vi "Television.vi"() -> ()   [LabVIEW 2021]
panel:
  in  "Mute":bool
  in  "Volume":dbl(knob) scale=0.0..100.0
  in  "off":bool
  in  "on":bool
  in  "channel2":bool
  in  "channel 1":bool
  in  "WindowsMediaPlayer":refnum<k7>(container)
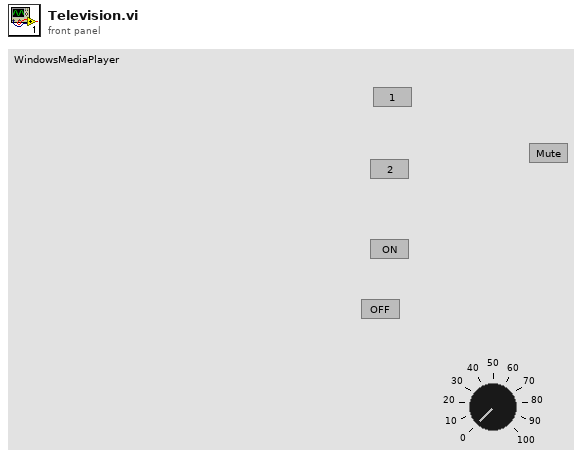
[diagram p1: front panel]
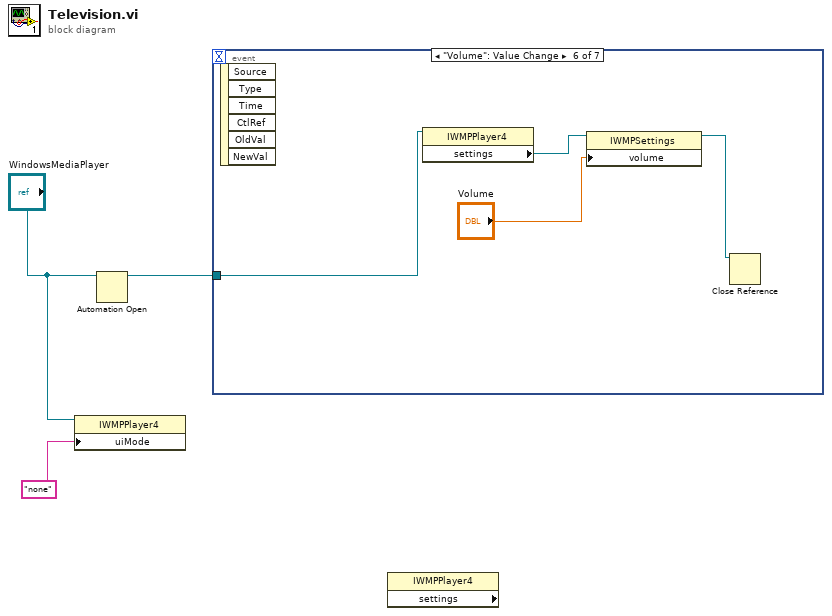
[diagram p0: block diagram]
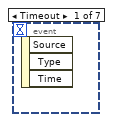
[diagram p2: hidden frame]
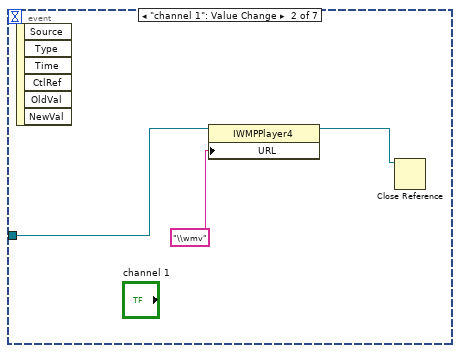
[diagram p3: hidden frame]
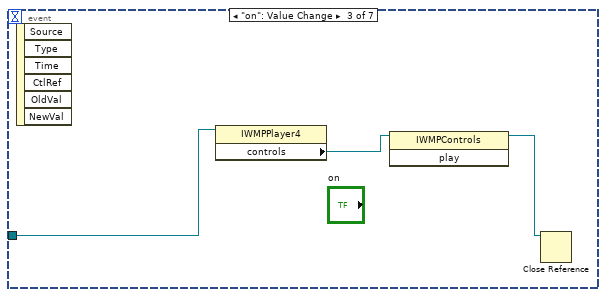
[diagram p4: hidden frame]
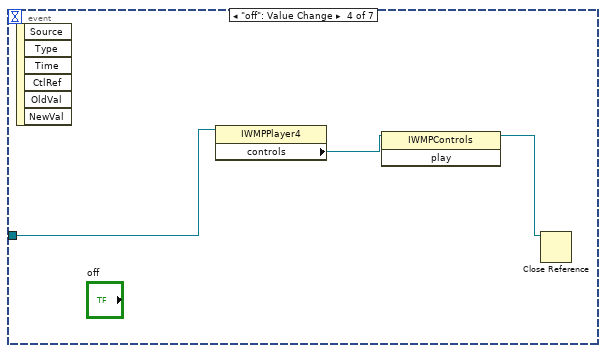
[diagram p5: hidden frame]
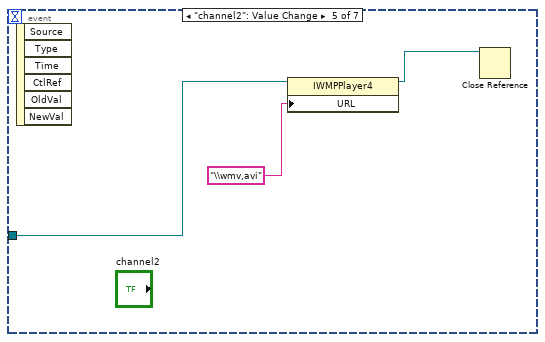
[diagram p6: hidden frame]
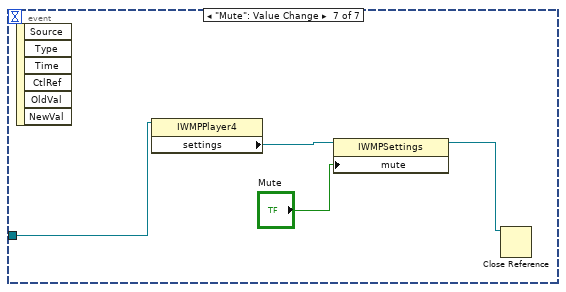
[diagram p7: hidden frame]
diagram:
  n1 = property class="IWMPPlayer4"(reference="WindowsMediaPlayer", "uiMode"="none") -> ()  [unwired: 1 in, 2 out]
  n2 = Automation Open(Automation Refnum="WindowsMediaPlayer") -> (Automation Refnum=w3:refnum<k7>)  [unwired: 3 in, 1 out]
  n3 = event shown="[5] \"Volume\": Value Change" {
    selector: _ -> [_ _ _ _ _ _ _]
    dyn-events: _ -> [_ _ _ _ _ _ _]
    timeout: _ -> [_ _ _ _ _ _ _]
    tunnel: w3 -> [_ w6 w9 w12 w15 w19 w23]
    event Timeout {
      n4 = event-data() -> ()  [unwired: 1 in, 3 out]
    }
    event "channel 1": Value Change {
      n5 = event-data() -> ()  [unwired: 1 in, 6 out]
      n6 = property class="IWMPPlayer4"(reference=w6, "URL"="\\wmv") -> (reference out=w4:refnum<k7>)  [unwired: 1 in, 1 out]
      n7 = Close Reference(reference=w4) -> ()  [unwired: 1 in, 1 out]
    }
    event "on": Value Change {
      n8 = event-data() -> ()  [unwired: 1 in, 6 out]
      n9 = property class="IWMPPlayer4"(reference=w9) -> ("controls"=w7:refnum<k7>)  [unwired: 1 in, 2 out]
      n10 = invoke class="IWMPControls" method="play"(reference=w7) -> (reference out=w8:refnum<k7>)  [unwired: 2 in, 2 out]
      n11 = Close Reference(reference=w8) -> ()  [unwired: 1 in, 1 out]
    }
    event "off": Value Change {
      n12 = event-data() -> ()  [unwired: 1 in, 6 out]
      n13 = property class="IWMPPlayer4"(reference=w12) -> ("controls"=w10:refnum<k7>)  [unwired: 1 in, 2 out]
      n14 = invoke class="IWMPControls" method="play"(reference=w10) -> (reference out=w11:refnum<k7>)  [unwired: 2 in, 2 out]
      n15 = Close Reference(reference=w11) -> ()  [unwired: 1 in, 1 out]
    }
    event "channel2": Value Change {
      n16 = event-data() -> ()  [unwired: 1 in, 6 out]
      n17 = property class="IWMPPlayer4"(reference=w15, "URL"="\\wmv,avi") -> (reference out=w14:refnum<k7>)  [unwired: 1 in, 1 out]
      n18 = Close Reference(reference=w14) -> ()  [unwired: 1 in, 1 out]
    }
    event "Volume": Value Change {
      n19 = event-data() -> ()  [unwired: 1 in, 6 out]
      n20 = property class="IWMPPlayer4"(reference=w19) -> ("settings"=w17:refnum<k7>)  [unwired: 1 in, 2 out]
      n21 = property class="IWMPSettings"(reference=w17, "volume"="Volume") -> (reference out=w18:refnum<k7>)  [unwired: 1 in, 1 out]
      n22 = Close Reference(reference=w18) -> ()  [unwired: 1 in, 1 out]
    }
    event "Mute": Value Change {
      n23 = event-data() -> ()  [unwired: 1 in, 6 out]
      n24 = property class="IWMPPlayer4"(reference=w23) -> ("settings"=w22:refnum<k7>)  [unwired: 1 in, 2 out]
      n25 = property class="IWMPSettings"(reference=w22, "mute"="Mute") -> (reference out=w20:refnum<k7>)  [unwired: 1 in, 1 out]
      n26 = Close Reference(reference=w20) -> ()  [unwired: 1 in, 1 out]
    }
  }
  n27 = property class="IWMPPlayer4" props=["settings"]() -> ()  [unwired: 2 in, 3 out]
